vi "Handle Error.vi"(8 "error in (no error)":errorcluster, 11 "Nested in":refnum<class "Nested.lvclass">) -> (0 "error out":errorcluster, 2 "stop actor?":bool=TRUE, 3 "Nested out":refnum<class "Nested.lvclass">)   [LabVIEW 2020, in "Nested.lvlib" / "Nested.lvclass"]
doc: "(<B>Filename</B>: Actor Framework.lvlib:Actor.lvclass:Handle Error.vi)\n\nDefines how the actor handles an error that occurred while processing a message. By default, this method does nothing except stop the actor."
uses:
  Nested.lvclass
  <vilib>/ActorFramework/Actor/Actor.lvclass
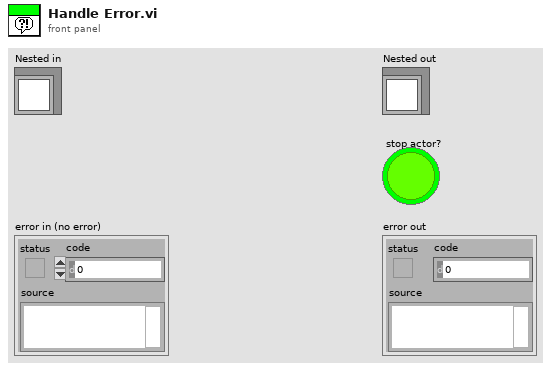
[diagram p1: front panel]
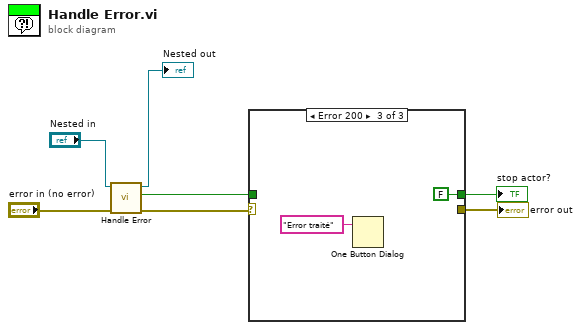
[diagram p0: block diagram]
diagram:
  n1 = call-parent "Handle Error.vi"("error in (no error)"="error in (no error)", "Actor in"="Nested in") -> ("error out"=w4:errorcluster, "stop actor?"=w3:bool, "Actor out"=→"Nested out":refnum<class "Nested.lvclass">)  [unwired: 7 in]
  n2 = case shown="Error 200" w4 {
    selector: w4 -> [w8 w10 _]
    tunnel: w3 -> [w9 w11 _]
    tunnel: [w9 w11 FALSE ("stop actor?")] -> w2
    tunnel: [w8 w10 _] -> w1
    frame No Error {
    }
    frame Default {
    }
    frame Error {
      n3 = One Button Dialog(message="Error traité") -> ()  [unwired: 1 in, 1 out]
    }
  }
  "stop actor?" <- w2
  "error out" <- w1
